vi "AWC Messen SP.vi"(11 "Samplepoint":u16) -> (3 "Anweisungscode":u16)   [LabVIEW 2020, in "PNS.lvlib"]
uses:
  PNS.lvlib
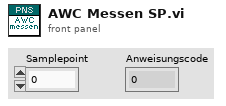
[diagram p1: front panel]
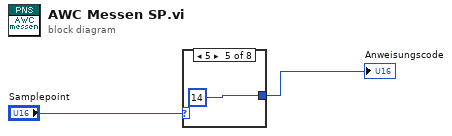
[diagram p0: block diagram]
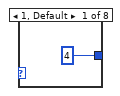
[diagram p2: hidden frame]
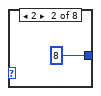
[diagram p3: hidden frame]
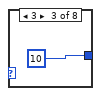
[diagram p4: hidden frame]
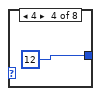
[diagram p5: hidden frame]
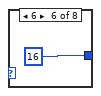
[diagram p6: hidden frame]
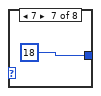
[diagram p7: hidden frame]
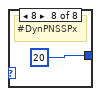
[diagram p8: hidden frame]
diagram:
  n1 = case shown="5" "Samplepoint" {
    tunnel: [u16 4 ("Anweisungscode") u16 8 ("Anweisungscode") u16 10 ("Anweisungscode") u16 12 ("Anweisungscode") u16 14 ("Anweisungscode") u16 16 ("Anweisungscode") u16 18 ("Anweisungscode") u16 20 ("Anweisungscode")] -> w2
    frame 1, Default {
    }
    frame 2 {
    }
    frame 3 {
    }
    frame 4 {
    }
    frame 5 {
    }
    frame 6 {
    }
    frame 7 {
    }
    frame 8 {
      # "#DynPNSSPx"
    }
  }
  "Anweisungscode" <- w2
